vi "Change Desired Temperature.vi"(8 "error in (no error)":errorcluster, 10 "Desired Temperature":dbl, 11 "Cooler Controller in":refnum<class "Cooler Controller.lvclass">) -> (0 "error out":errorcluster, 3 "Cooler Controller out":refnum<class "Cooler Controller.lvclass">)   [LabVIEW 2018, in "Cooler Controller.lvlib" / "Cooler Controller.lvclass"]
doc: "Change the desired temperature of the cooling system."
uses:
  Cooler Controller.lvclass
  Cooler Controller.lvclass/Cooler Controller.ctl
  Cooler/Write Desired Temperature Msg/Write Desired Temperature Msg.lvclass/Write Desired Temperature Msg.ctl
  <vilib>/ActorFramework/Message Enqueuer/Message Enqueuer.lvclass/Message Enqueuer.ctl
  <vilib>/ActorFramework/Message Enqueuer/Enqueue.vi
  Cooler/Write Desired Temperature Msg/Write Desired Temperature Msg.lvclass
  C:/Program Files (x86)/National Instruments/LabVIEW 2018/vi.lib/ActorFramework/Message/Message.lvclass
  <vilib>/ActorFramework/Message Priority Queue/Priority Enqueue.vi
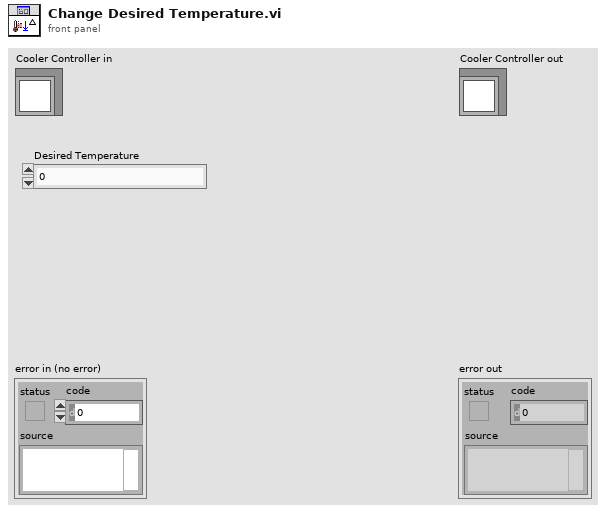
[diagram p1: front panel]
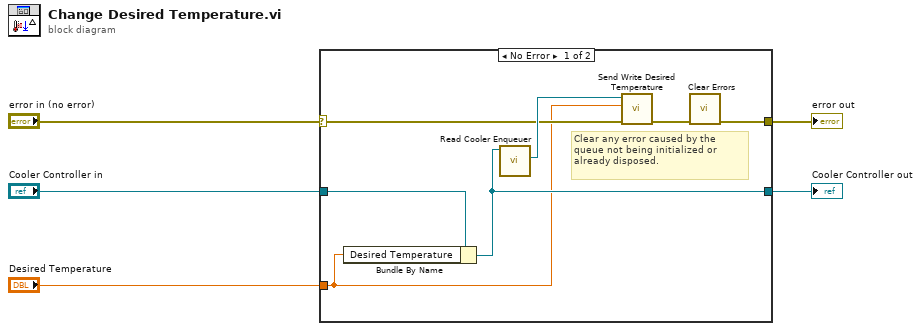
[diagram p0: block diagram]
diagram:
  n1 = case shown="No Error" "error in (no error)" {
    selector: "error in (no error)" -> [w11 w14]
    tunnel: [w6 w14] -> w4
    tunnel: [w9 w13] -> w2
    tunnel: "Cooler Controller in" -> [w10 w13]
    tunnel: "Desired Temperature" -> [w8 _]
    frame No Error {
      # "Clear any error caused by the queue not being initialized or already disposed."
      n2 = Bundle By Name(cluster=w10, "Desired Temperature"=w8) -> (w9:refnum<class "Cooler Controller.lvclass">)
      n3 = call "Read Cooler Enqueuer.vi"("Cooler Controller"=w9) -> ("Cooler Enqueuer"=w12:refnum<class "Message Enqueuer.lvclass">)  [unwired: 10 in]
      n4 = call "Send Write Desired Temperature.vi"("error in (no error)"=w11, "Desired Temperature"=w8, "Message Enqueuer"=w12) -> ("error out"=w7:errorcluster)  [unwired: 8 in]
      n5 = call <vilib>:"Clear Errors.vi"("error in (no error)"=w7) -> ("error out"=w6:errorcluster)  [unwired: 5 in, 1 out]
    }
    frame Error {
    }
  }
  "error out" <- w4
  "Cooler Controller out" <- w2
